vi "rad_Apply Network Settings (DHCP).bak.vi"(6 "Timeout in ms (4s)":u32=4000, 8 "error in (no error)":errorcluster, 10 "Requested settings":T1={"Hostname"="", "Serial number"="", "Product name"="", "Product code"=0, "System status"="", "Credential type"=enum."None/Unlocked", "User added?"=FALSE, "Primary NIC"={"MAC address"="", "IP Address Request Mode"=2, "IP address"="", "Subnet mask"="", "Gateway"="", "DNS server"=""}} {"Primary NIC"."IP Address Request Mode" items=["Static"=1, "DHCP/Link-Local"=2, "Link-Local Only"=4, "DHCP Only"=8]}, 11 "Existing settings":T1={"Hostname"="", "Serial number"="", "Product name"="", "Product code"=0, "System status"="", "Credential type"=enum."None/Unlocked", "User added?"=FALSE, "Primary NIC"={"MAC address"="", "IP Address Request Mode"=2, "IP address"="", "Subnet mask"="", "Gateway"="", "DNS server"=""}} {"Primary NIC"."IP Address Request Mode" items=["Static"=1, "DHCP/Link-Local"=2, "Link-Local Only"=4, "DHCP Only"=8]}) -> (0 "error out":errorcluster, 3 "Target settings out":T1={"Hostname"="", "Serial number"="", "Product name"="", "Product code"=0, "System status"="", "Credential type"=enum."None/Unlocked", "User added?"=FALSE, "Primary NIC"={"MAC address"="", "IP Address Request Mode"=2, "IP address"="", "Subnet mask"="", "Gateway"="", "DNS server"=""}} {"Primary NIC"."IP Address Request Mode" items=["Static"=1, "DHCP/Link-Local"=2, "Link-Local Only"=4, "DHCP Only"=8]})   [LabVIEW 2013]
uses:
  TypeDefs/rad_Target Information.ctl
  TypeDefs/rad_Target Network Settings.ctl
  <vilib>/nisyscfg/Save Changes (System).vi
  <vilib>/nisyscfg/Close (System).vi
  <vilib>/nisyscfg/nisyscfg.lvlib
  <resource>/objmgr/nisysapi.rc
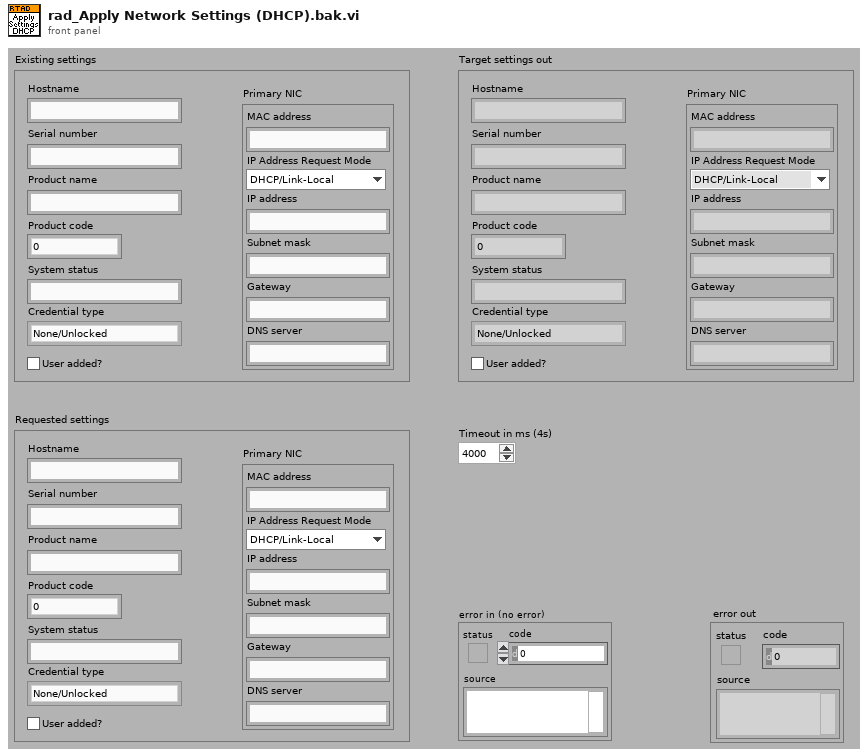
[diagram p1: front panel]
types:
  T1 = typedef "rad_Target Information.ctl" = cluster{"Hostname":string, "Serial number":string, "Product name":string, "Product code":i32, "System status":string, "Credential type":enum16{"None/Unlocked", "FTP Password", "NIAuth Credentials"}, "User added?":bool, "Primary NIC":T2}
  T2 = typedef "rad_Target Network Settings.ctl" = cluster{"MAC address":string, "IP Address Request Mode":i32, "IP address":string, "Subnet mask":string, "Gateway":string, "DNS server":string}
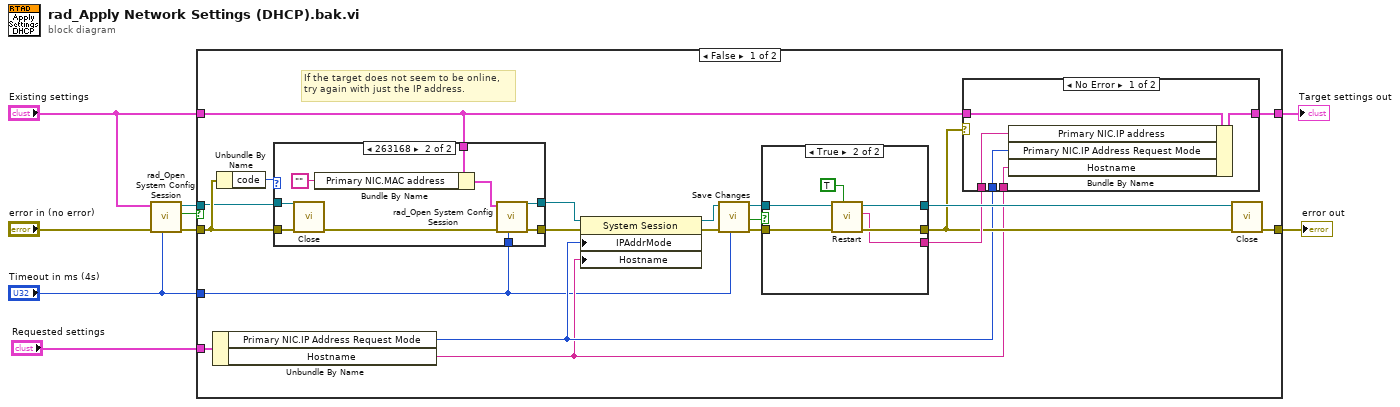
[diagram p0: block diagram]
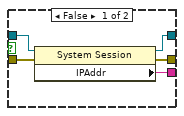
[diagram p4: hidden frame]
diagram:
  n1 = call "rad_Open System Config Session.vi"("Timeout ms (4000)"="Timeout in ms (4s)", "error in (no error)"="error in (no error)", "Target settings"="Existing settings") -> ("error out"=w6:errorcluster, "Cancelled"=w4:bool, "Session out"=w7:refnum<k21>)  [unwired: 5 in, 1 out]
  n2 = case shown="False" w4 {
    tunnel: w7 -> [w14 _]
    tunnel: w6 -> [w15 w59]
    tunnel: [w29 w59] -> w8
    tunnel: "Timeout in ms (4s)" -> [w10 _]
    tunnel: "Existing settings" -> [w11 w58]
    tunnel: [w23 w58] -> w3
    tunnel: "Requested settings" -> [w19 _]
    frame False {
      # "If the target does not seem to be online,\ntry again with just the IP address."
      n3 = Unbundle By Name(w19) -> ("Primary NIC.IP Address Request Mode"=w18:i32, "Hostname"=w17:string)
      n4 = Unbundle By Name(w15) -> ("code"=w16:i32)
      n5 = case shown="263168" w16 {
        tunnel: w15 -> [w30 w40]
        tunnel: w14 -> [w31 w39]
        tunnel: w11 -> [_ w38]
        tunnel: w10 -> [_ w34]
        tunnel: [w30 w33] -> w13
        tunnel: [w31 w32] -> w12
        frame Default {
        }
        frame 263168 {
          n6 = call-poly <vilib>:"Close.vi"("error in (no error)"=w40, "Session in"=w39) -> ("error out"=w35:errorcluster)  [unwired: 9 in]
          n7 = Bundle By Name(cluster=w38, "Primary NIC.MAC address"="") -> (w36:T1)
          n8 = call "rad_Open System Config Session.vi"("Timeout ms (4000)"=w34, "error in (no error)"=w35, "Target settings"=w36) -> ("error out"=w33:errorcluster, "Session out"=w32:refnum<k21>)  [unwired: 5 in, 2 out]
        }
      }
      n9 = property class="System Session"(reference=w12, error in=w13, "IPAddrMode"=w18, "Hostname"=w17) -> (reference out=w28:refnum<k21>, error out=w27:errorcluster)
      n10 = call-poly <vilib>:"Save Changes.vi"("Remote Timeout (300,000 ms)"=w10, "error in (no error)"=w27, "Session in"=w28) -> ("error out"=w25:errorcluster, "Changes Require Restart"=w26:bool, "Session out"=w24:refnum<k21>)  [unwired: 5 in, 1 out]
      n11 = case shown="True" w26 {
        tunnel: w25 -> [w51 w57]
        tunnel: [w50 w56] -> w20
        tunnel: w24 -> [w49 w55]
        tunnel: [w48 w54] -> w22
        tunnel: [w47 w52] -> w21
        frame False {
          n12 = property class="System Session"(reference=w49, error in=w51) -> (reference out=w48:refnum<k21>, error out=w50:errorcluster, "IPAddr"=w47:string)
        }
        frame True {
          n13 = call <vilib>:"Restart.vi"("Wait Until Complete (T)"=TRUE ("wait until complete (T)"), "error in (no error)"=w57, "Session in"=w55) -> ("error out"=w56:errorcluster, "New IP Address"=w52:string, "Session out"=w54:refnum<k21>)  [unwired: 6 in]
        }
      }
      n14 = case shown="No Error" w20 {
        tunnel: w11 -> [w45 w46]
        tunnel: [w44 w46] -> w23
        tunnel: w17 -> [w43 _]
        tunnel: w18 -> [w42 _]
        tunnel: w21 -> [w41 _]
        frame No Error {
          n15 = Bundle By Name(cluster=w45, "Primary NIC.IP address"=w41, "Primary NIC.IP Address Request Mode"=w42, "Hostname"=w43) -> (w44:T1)
        }
        frame Error {
        }
      }
      n16 = call-poly <vilib>:"Close.vi"("error in (no error)"=w20, "Session in"=w22) -> ("error out"=w29:errorcluster)  [unwired: 9 in]
    }
    frame True {
    }
  }
  "error out" <- w8
  "Target settings out" <- w3
